vi "OP300ZP_prep bdd Vpack.vi"(8 "tabin":string[](array[string]), 11 "OCV":string) -> (0 "tabout":string[](array[string]))   [LabVIEW 2020]
uses:
  OP300ZP_selectdata.ctl
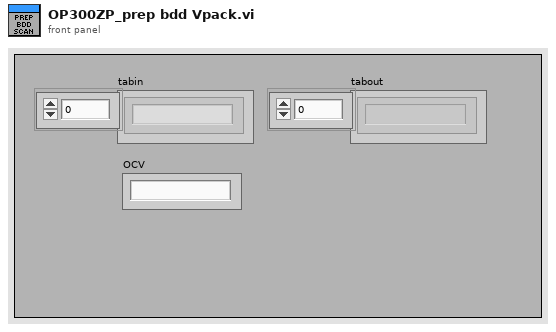
[diagram p1: front panel]
types:
  T1 = typedef "OP300ZP_selectdata.ctl" = u16
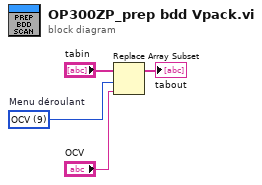
[diagram p0: block diagram]
diagram:
  w2 = T1 9 items=["IdOp300", "DateStart", "DeltaTC", "DeltaVC", "ImageVers", "IniFileVers", "InsuN", "InsuP", "MCU", "OCV", "Operateur", "Pass", "SN", "SoftVers", "TC0", "TC1", "TempsTest", "Tfactory", "Type", "VC0", "VC1"]  # Menu déroulant
  n1 = Replace Array Subset(array="tabin", new element="OCV", index=w2) -> (→"tabout":string[])
